vi "labcontrol.vi"(9 "IP address":string="192.168.4.129", 10 "Enum":T2(ring), 11 "data":T1(array[cluster])) -> (1 "command_debug":string, 2 "error out":errorcluster, 3 "data out":string)   [LabVIEW 2014]
uses:
  RedPitaya/RedPitaya.lvlib
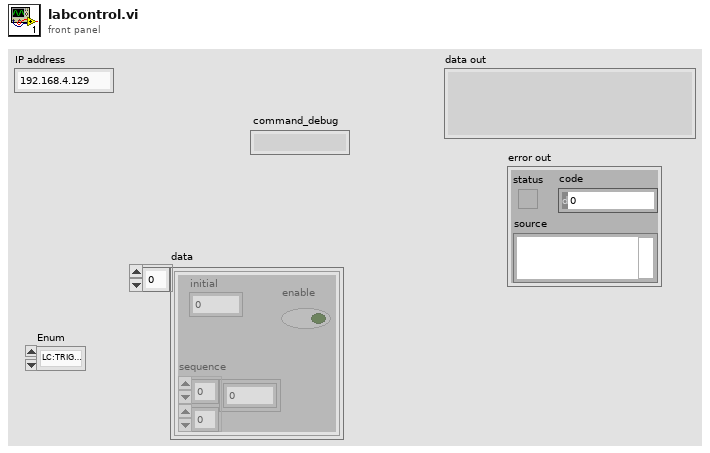
[diagram p1: front panel]
types:
  T1 = cluster{"sequence":dbl[][], "initial":dbl, "enable":bool}[]
  T2 = enum16{"LC:TRIG:SOFT", "LC:TRIG:AWAIT", "LC:DATA"}
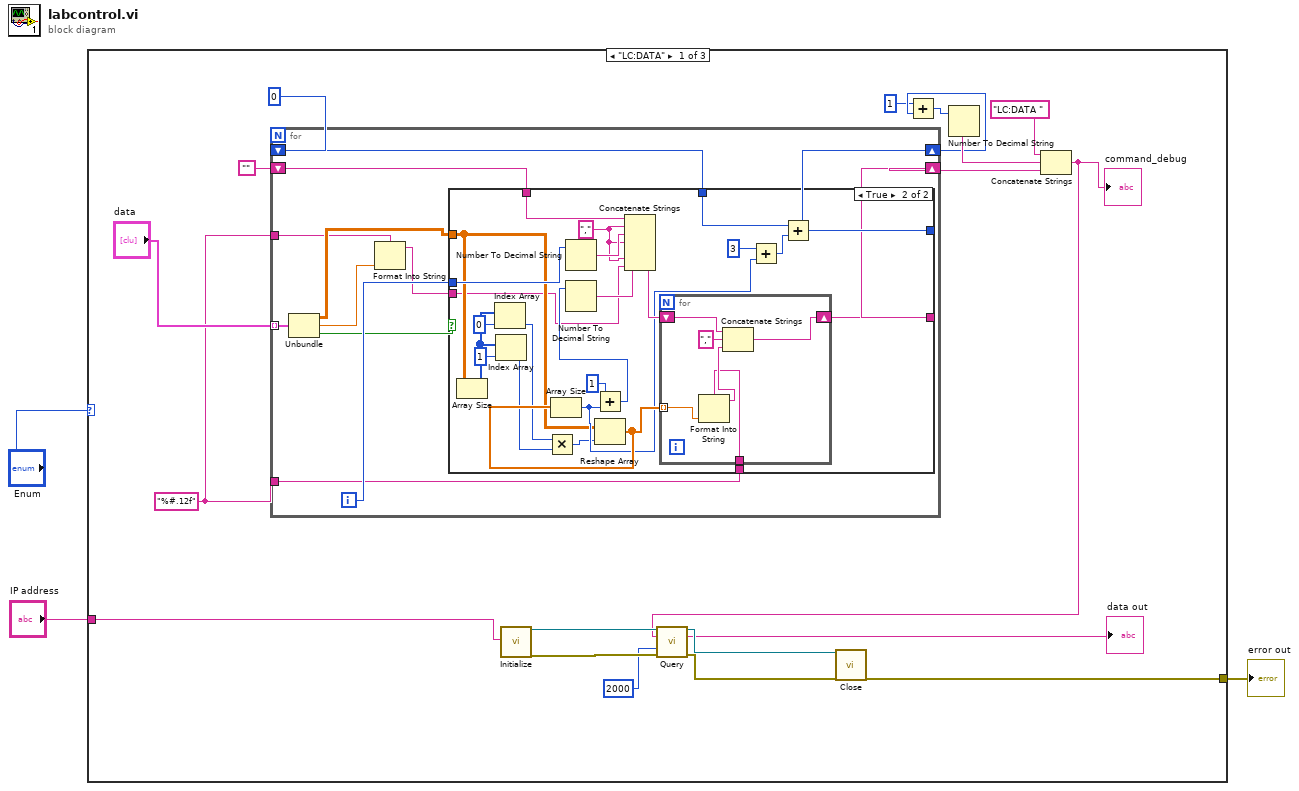
[diagram p0: block diagram]
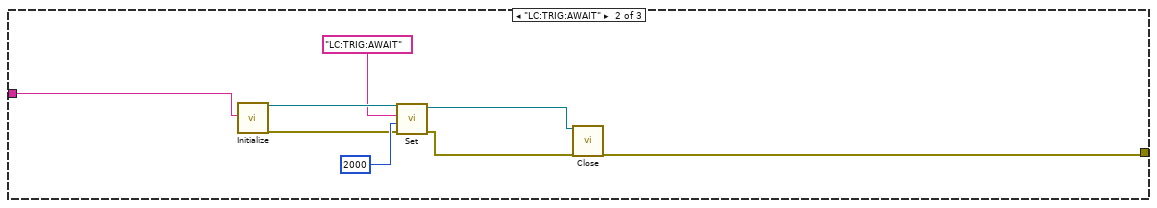
[diagram p3: hidden frame]
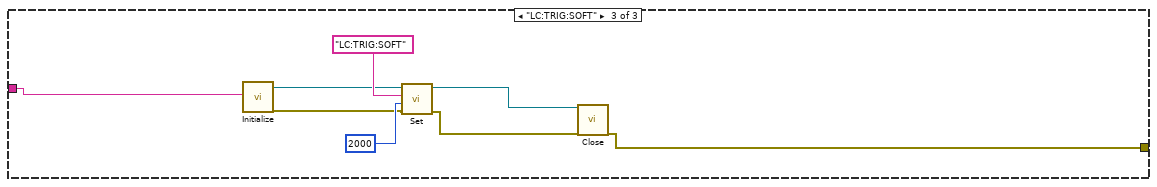
[diagram p4: hidden frame]
diagram:
  n1 = case shown="\"LC:DATA\"" "Enum" {
    tunnel: "IP address" -> [w12 w74 w82]
    tunnel: [w11 w73 w81] -> w1
    frame "LC:DATA" {
      w4 = "%#.12f" ("format string")
      n2 = for {
        shift-right: [w31] -> w8
        shift-left: 0 -> [w32]
        shift-right: [w30] -> w20
        shift-left: "" -> [w34]
        tunnel: "data" -> [w29] mode=indexing
        tunnel: w4 -> [w24]
        tunnel: w4 -> [w23]
        i -> [w33]
        n3 = Unbundle(w29) -> ("sequence"=w27:dbl[][], "initial"=w25:dbl, "enable"=w28:bool)
        n4 = Format Into String(format string=w24, w25) -> (resulting string=w26:string)  [unwired: 2 in, 1 out]
        n5 = case shown="True" w28 {
          tunnel: w27 -> [_ w45]
          tunnel: w34 -> [w35 w60]
          tunnel: w33 -> [_ w58]
          tunnel: w26 -> [_ w38]
          tunnel: w32 -> [w36 w51]
          tunnel: [w36 w47] -> w31
          tunnel: [w35 w46] -> w30
          tunnel: w23 -> [_ w37]
          frame False {
          }
          frame True {
            w55 = "," ("string")
            n6 = Array Size(array=w45) -> (size(s)=w43:i32[])
            n7 = Index Array(array=w43, index=0) -> (element=w40:i32)
            n8 = Index Array(array=w43, index=1) -> (element=w39:i32)
            n9 = Multiply(x=w40, y=w39) -> (x*y=w44:i32)
            n10 = Number To Decimal String(number=w58) -> (decimal integer string=w59:string)  [unwired: 1 in]
            n11 = Reshape Array(w45, w44) -> (w54:dbl[])
            n12 = Array Size(array=w54) -> (size(s)=w49:i32)
            n13 = Add(x=1, y=w49) -> (x+y=w53:i32)
            n14 = Number To Decimal String(number=w53) -> (decimal integer string=w56:string)  [unwired: 1 in]
            n15 = Concatenate Strings(w60, w55, w59, w55, w56, w55, w38) -> (w57:string)
            n16 = for {
              tunnel: w54 -> [w62] mode=indexing
              shift-right: [w64] -> w46
              shift-left: w57 -> [w65]
              tunnel: w37 -> [w61]
              n17 = Format Into String(format string=w61, w62) -> (resulting string=w63:string)  [unwired: 2 in, 1 out]
              n18 = Concatenate Strings(w65, "," ("string"), w63) -> (w64:string)
            }
            n19 = Add(x=3, y=w49) -> (x+y=w50:i32)
            n20 = Add(x=w51, y=w50) -> (x+y=w47:i32)
          }
        }
      }
      n21 = call "Initialize.vi"("IP address"=w12) -> ("RedPitaya TCP Connection"=w17:refnum<k5>, "error out"=w18:errorcluster)  [unwired: 17 in]
      n22 = Add(x=1, y=w8) -> (x+y=w9:i32)
      n23 = Number To Decimal String(number=w9) -> (decimal integer string=w19:string)  [unwired: 1 in]
      n24 = Concatenate Strings("LC:DATA " ("string"), w19, w20) -> (w10:string)
      "command_debug" <- w10
      n25 = call "Query.vi"("RedPitaya connection in"=w17, "SCPI Query"=w10, "timeout ms (2000)"=2000, "error in"=w18) -> ("RedPitaya connection out"=w14:refnum<k5>, "data out"=→"data out":string, "error out"=w13:errorcluster)  [unwired: 9 in]
      n26 = call "Close.vi"("connection ID"=w14, "error in"=w13) -> ("error out"=w11:errorcluster)  [unwired: 17 in]
    }
    frame "LC:TRIG:AWAIT" {
      n27 = call "Initialize.vi"("IP address"=w74) -> ("RedPitaya TCP Connection"=w72:refnum<k5>, "error out"=w69:errorcluster)  [unwired: 17 in]
      n28 = call "Set.vi"("error in"=w69, "timeout ms (2000)"=2000, "SCPI Message"="LC:TRIG:AWAIT" ("SCPI Query"), "RedPitaya connection in"=w72) -> ("error out"=w68:errorcluster, "RedPitaya connection out"=w67:refnum<k5>)  [unwired: 5 in, 1 out]
      n29 = call "Close.vi"("connection ID"=w67, "error in"=w68) -> ("error out"=w73:errorcluster)  [unwired: 17 in]
    }
    frame "LC:TRIG:SOFT" {
      n30 = call "Initialize.vi"("IP address"=w82) -> ("RedPitaya TCP Connection"=w75:refnum<k5>, "error out"=w78:errorcluster)  [unwired: 17 in]
      n31 = call "Set.vi"("error in"=w78, "timeout ms (2000)"=2000, "SCPI Message"="LC:TRIG:SOFT" ("SCPI Query"), "RedPitaya connection in"=w75) -> ("error out"=w77:errorcluster, "RedPitaya connection out"=w76:refnum<k5>)  [unwired: 5 in, 1 out]
      n32 = call "Close.vi"("connection ID"=w76, "error in"=w77) -> ("error out"=w81:errorcluster)  [unwired: 17 in]
    }
  }
  "error out" <- w1
